vi "HumanPulse Detector.vi"() -> ()   [LabVIEW 2015]
uses:
  <vilib>/measure/mamon.llb/Waveform Peak Detection for N Chan.vi
  <vilib>/measure/NI_MAPro.lvlib
  <vilib>/Analysis/NI_AAL_SigProc.lvlib
panel:
  in  "peaks/valleys":u16(ring) items=["Peaks", "Valleys"]
  in  "stop (F)":bool
  out "LED Voltage":dbl
  out "Max x 0.7":dbl
  out "Filtered Signal":dynamicdata(graph)
  out "Acquired Raw Signal":dynamicdata(graph)
  out "Max":dbl
  out "\"Heart Rate\" (BPM)":dbl
  out "Frequency (Hz)":dbl
  out "Scalar":dbl
  # "Human Pulse Detector"
  # "by Anni Blair, Edith Acosta, Kris Bickham"
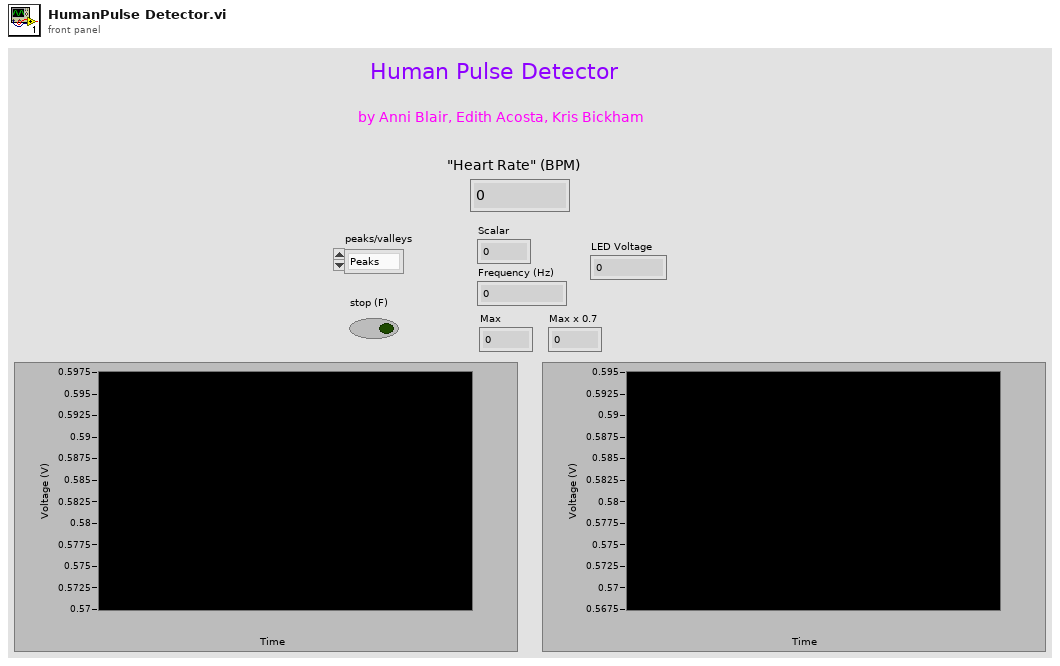
[diagram p1: front panel]
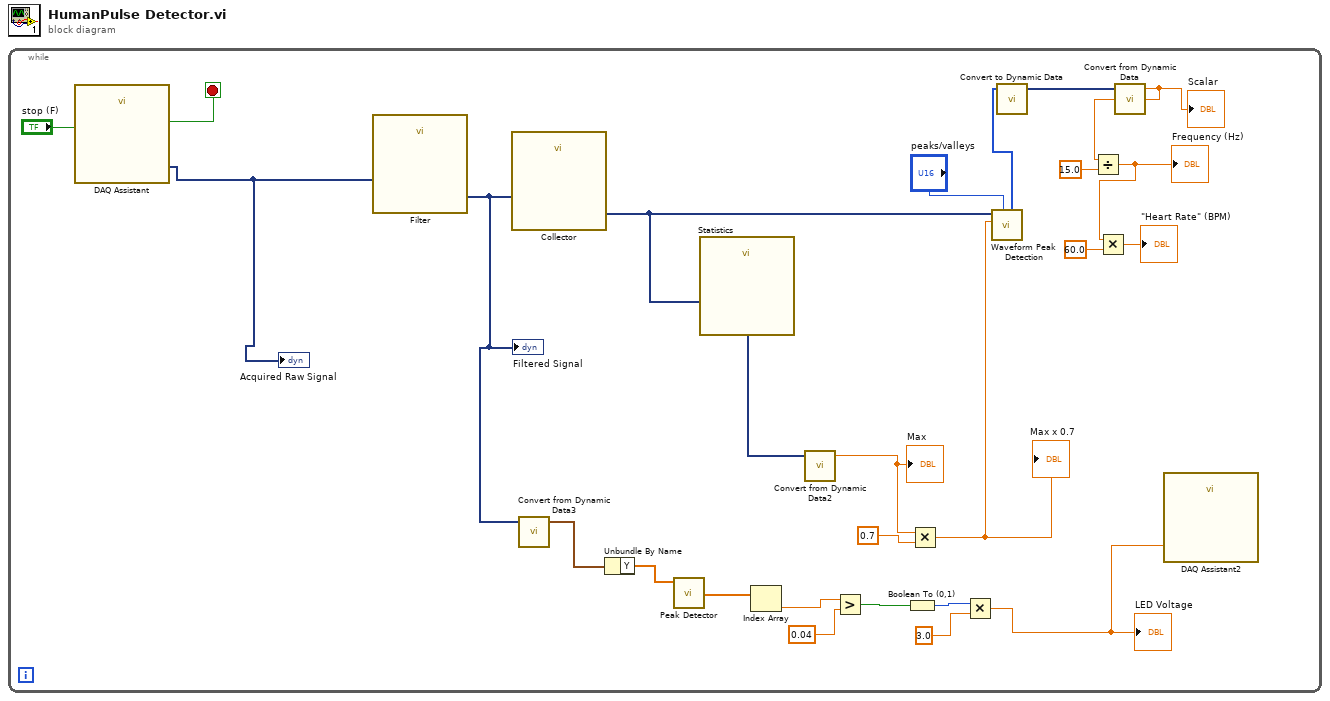
[diagram p0: block diagram]
diagram:
  n1 = while {
    stop <- w25 stop-if-true
    n2 = call "DAQ Assistant"("stop (F)"="stop (F)") -> ("data"=w2:dynamicdata, "stopped"=w25:bool)  [unwired: 15 in, 2 out]
    "Acquired Raw Signal" <- w2
    n3 = call "Filter"("Signal"=w2) -> ("Filtered Signal"=w24:dynamicdata)  [unwired: 2 in, 8 out]
    "Filtered Signal" <- w24
    n4 = call "Collector"("Signals"=w24) -> ("Collected Signals"=w12:dynamicdata)  [unwired: 9 in, 1 out]
    n5 = call "Convert from Dynamic Data3"("Dynamic Data Type"=w24) -> ("Waveform"=w17:waveform(dbl))  [unwired: 1 in, 2 out]
    n6 = Unbundle By Name(w17) -> ("Y"=w16:dbl[])
    n7 = call <vilib>:"Peak Detector.vi"("X"=w16) -> ("Amplitudes"=w23:dbl[])  [unwired: 6 in, 4 out]
    n8 = call "Statistics"("Signals"=w12) -> ("Maximum"=w11:dynamicdata)  [unwired: 23 in, 3 out]
    n9 = Index Array(array=w23) -> (element=w20:dbl)  [unwired: 1 in]
    n10 = call "Convert from Dynamic Data2"("Dynamic Data Type"=w11) -> ("Scalar"=w13:dbl)  [unwired: 3 in]
    "Max" <- w13
    n11 = Greater?(x=w20, y=0.04) -> (0:w21:bool)
    n12 = Boolean To (0,1)(Boolean=w21) -> (0, 1=w22:i16)
    n13 = Multiply(x=w13, y=0.7) -> (x*y=w15:dbl)
    "Max x 0.7" <- w15
    n14 = Multiply(x=w22, y=3.0) -> (x*y=w3:dbl)
    "LED Voltage" <- w3
    n15 = call-poly <vilib>:"Waveform Peak Detection.vi"("peaks/valleys"="peaks/valleys", "threshold"=w15, "Signals In"=w12) -> ("# found"=w5:i32[])  [unwired: 4 in, 4 out]
    n16 = call "Convert to Dynamic Data"("Array"=w5) -> ("Dynamic Data Type"=w6:dynamicdata)  [unwired: 3 in]
    n17 = call "Convert from Dynamic Data"("Dynamic Data Type"=w6) -> ("Scalar"=w4:dbl)  [unwired: 3 in]
    "Scalar" <- w4
    n18 = Divide(x=w4, y=15.0) -> (x/y=w8:dbl)
    "Frequency (Hz)" <- w8
    n19 = Multiply(x=w8, y=60.0) -> (x*y=→"\"Heart Rate\" (BPM)":dbl)
    n20 = call "DAQ Assistant2"("data"=w3) -> ()  [unwired: 17 in, 2 out]
  }
